vi "4461.Trigger.vi"(8 "error in (no error)":errorcluster, 11 "Instrument.Lockin in":refnum<class "Instrument.Lockin.lvclass">) -> (0 "error out":errorcluster, 3 "Instrument.Lockin out":refnum<class "Instrument.Lockin.lvclass">)   [LabVIEW 2016, in "LockinDAQ.lvclass"]
uses:
  LockinDAQ.lvclass
  <resource>/objmgr/daqmx.rc
  Typedefs/DAQType-enum.ctl
  <vilib>/DAQmx/configure/trigger.llb/DAQmx Start Trigger (Digital Edge).vi
  Instrument.Lockin/Instrument.Lockin.lvclass
  C:/Program Files (x86)/National Instruments/LabVIEW 2016/user.lib/LevyLab/Levylab Instruments/SMOs/Instrument/Instrument.lvclass
  C:/Program Files (x86)/National Instruments/LabVIEW 2016/user.lib/LevyLab/Levylab Instruments/SMOs/LevyLab/LevyLab.lvclass
  C:/Program Files (x86)/National Instruments/LabVIEW 2016/vi.lib/JKI/JKI SMO/SMO/SMO.lvclass
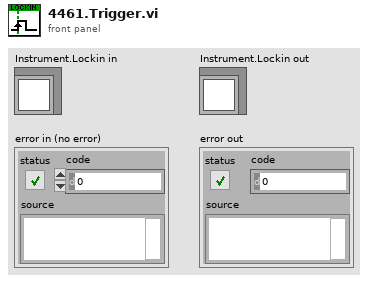
[diagram p1: front panel]
types:
  T1 = typedef "LockinDAQ.lvclass/DAQType-enum.ctl" = enum16{"None", "USB 4431", "PXI 446x"}
  T2 = cluster{"DAQ Type":T1, "master task":refnum<k21>, "RefClk.Src":tag, "SyncPulse.Src":tag, "Trigger.Src":tag, "SyncPulse.SyncTime":dbl}
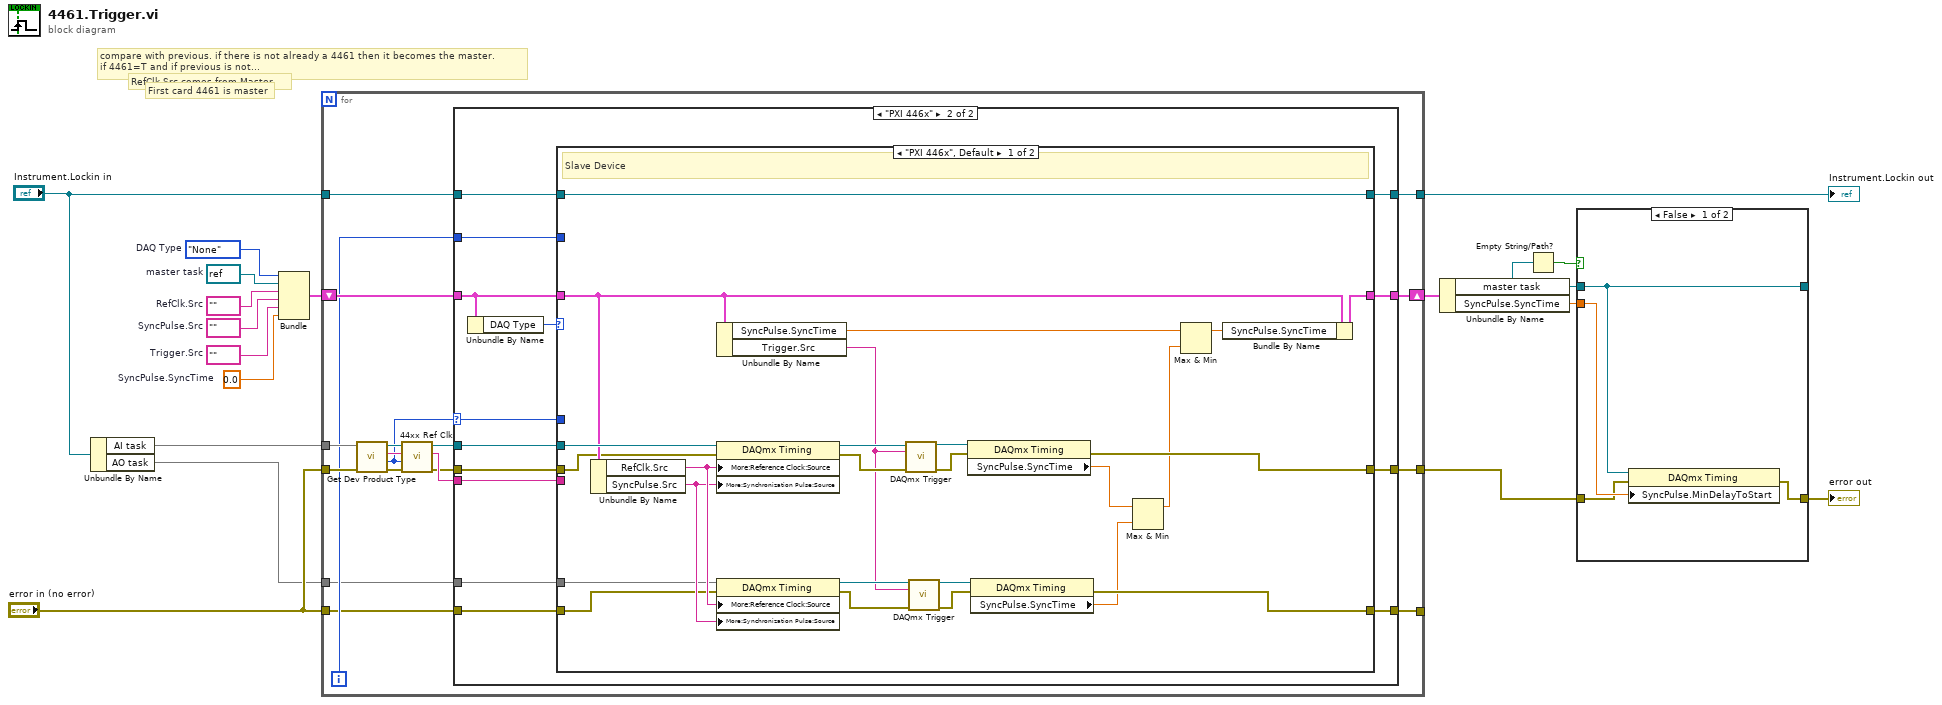
[diagram p0: block diagram]
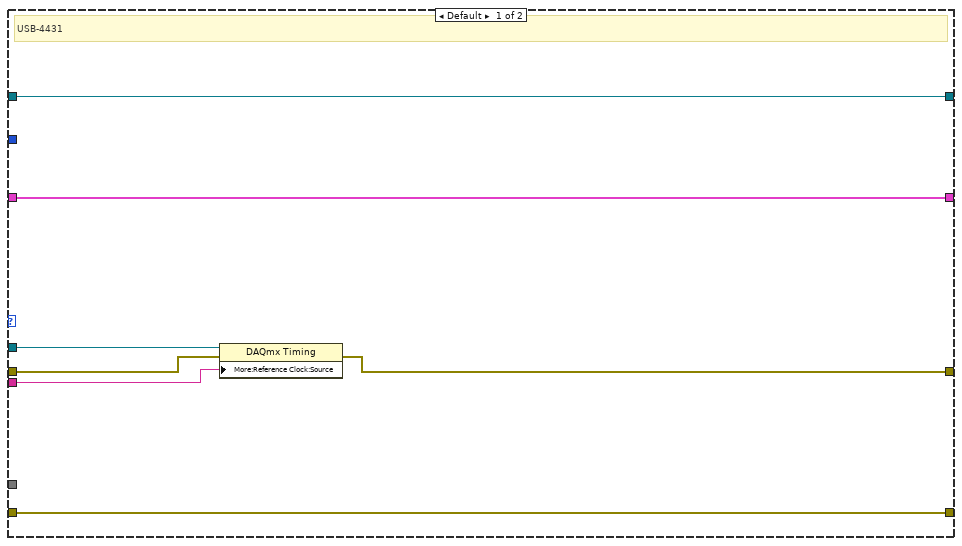
[diagram p2: hidden frame]
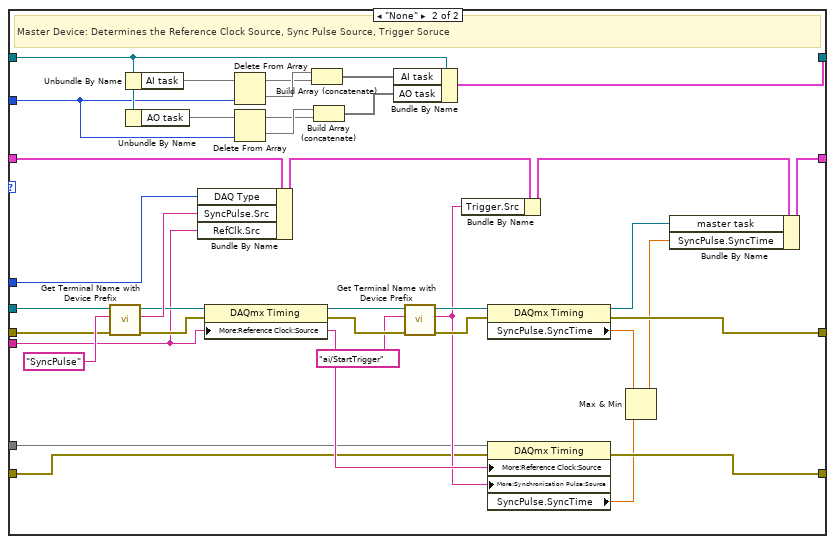
[diagram p3: hidden frame]
diagram:
  w2 = refnum<k21> refnum  # master task
  w12 = 0.0  # SyncPulse.SyncTime
  w11 = tag ""  # Trigger.Src
  w10 = tag ""  # SyncPulse.Src
  w3 = tag ""  # RefClk.Src
  w1 = DAQType-enum."None"  # DAQ Type
  # "RefClk.Src comes from Master"
  # "compare with previous. if there is not already a 4461 then it becomes the master. \nif 4461=T and if previous is not..."
  # "First card 4461 is master"
  n1 = Unbundle By Name("Instrument.Lockin in") -> ("AI task"=w6, "AO task"=w4)
  n2 = Bundle("DAQ Type"=w1, "master task"=w2, "RefClk.Src"=w3, "SyncPulse.Src"=w10, "Trigger.Src"=w11, "SyncPulse.SyncTime"=w12) -> (w9:T2)  [unwired: 1 in]
  n3 = for {
    tunnel: w6 -> [w36]
    tunnel: "error in (no error)" -> [w32]
    shift-right: [w27] -> w13
    shift-left: w9 -> [w30]
    tunnel: [w25] -> w17
    tunnel: "Instrument.Lockin in" -> [w24]
    tunnel: [w22] -> w7
    tunnel: [w21] -> _
    tunnel: "error in (no error)" -> [w20]
    tunnel: w4 -> [w19]
    i -> [w23]
    n4 = call "Get Dev Product Type.vi"("error in (no error)"=w32, "Refnum in"=w36) -> ("error out"=w35:errorcluster, "DAQ Type"=w31:T1, "ActiveDev"=w34:tag, "Refnum out"=w33:refnum<k21>)  [unwired: 6 in]
    n5 = call "44xx Ref Clk.vi"("error in (no error)"=w35, "DAQ Type"=w31, "ActiveDev"=w34, "Refnum in"=w33) -> ("error out"=w26:errorcluster, "RefClk.Src"=w28:tag, "Refnum out"=w29:refnum<k21>)  [unwired: 5 in]
    n6 = case shown="\"PXI 446x\"" w31 {
      selector: w31 -> [_ w54]
      tunnel: w30 -> [w43 w55]
      tunnel: w29 -> [w42 w57]
      tunnel: w28 -> [w41 w56]
      tunnel: [w43 w53] -> w27
      tunnel: w26 -> [w40 w52]
      tunnel: [w39 w51] -> w25
      tunnel: w24 -> [w38 w49]
      tunnel: w23 -> [_ w48]
      tunnel: [w38 w47] -> w22
      tunnel: [w37 w44] -> w21
      tunnel: w20 -> [w37 w46]
      tunnel: w19 -> [_ w45]
      frame Default {
        # "USB-4431"
        n7 = property class="DAQmx Timing"(reference=w42, error in=w40, "More:Reference Clock:Source"=w41) -> (error out=w39:errorcluster)  [unwired: 1 out]
      }
      frame "PXI 446x" {
        n8 = Unbundle By Name(w55) -> ("DAQ Type"=w50:T1)
        n9 = case shown="\"PXI 446x\", Default" w50 {
          tunnel: w57 -> [w82 w119]
          tunnel: w56 -> [_ w96]
          tunnel: w55 -> [w79 w118]
          tunnel: w54 -> [_ w117]
          tunnel: [w78 w106] -> w53
          tunnel: w52 -> [w65 w114]
          tunnel: [w76 w105] -> w51
          tunnel: w49 -> [w75 w91]
          tunnel: w48 -> [_ w90]
          tunnel: [w75 w97] -> w47
          tunnel: w46 -> [w64 w93]
          tunnel: w45 -> [w72 w94]
          tunnel: [w63 w92] -> w44
          frame "PXI 446x", Default {
            # "Slave Device"
            n10 = Unbundle By Name(w79) -> ("RefClk.Src"=w74:tag, "SyncPulse.Src"=w73:tag)
            n11 = Unbundle By Name(w79) -> ("SyncPulse.SyncTime"=w60:dbl, "Trigger.Src"=w68:tag)
            n12 = property class="DAQmx Timing"(reference=w82, error in=w65, "More:Reference Clock:Source"=w74, "More:Synchronization Pulse:Source"=w73) -> (reference out=w81:refnum<k21>, error out=w69:errorcluster)
            n13 = property class="DAQmx Timing"(reference=w72, error in=w64, "More:Reference Clock:Source"=w74, "More:Synchronization Pulse:Source"=w73) -> (reference out=w70:refnum<k21>, error out=w67:errorcluster)
            n14 = call-poly <vilib>:"DAQmx Trigger.vi"("task/channels in"=w81, "source"=w68, "error in"=w69) -> ("task out"=w80:refnum<k21>, "error out"=w77:errorcluster)  [unwired: 11 in]
            n15 = call-poly <vilib>:"DAQmx Trigger.vi"("task/channels in"=w70, "source"=w68, "error in"=w67) -> ("task out"=w71:refnum<k21>, "error out"=w66:errorcluster)  [unwired: 11 in]
            n16 = property class="DAQmx Timing"(reference=w80, error in=w77) -> (error out=w76:errorcluster, "SyncPulse.SyncTime"=w58:dbl)  [unwired: 1 out]
            n17 = property class="DAQmx Timing"(reference=w71, error in=w66) -> (error out=w63:errorcluster, "SyncPulse.SyncTime"=w62:dbl)  [unwired: 1 out]
            n18 = Max & Min(x=w58, y=w62) -> (max(x,y)=w61:dbl)  [unwired: 1 out]
            n19 = Max & Min(x=w60, y=w61) -> (max(x,y)=w59:dbl)  [unwired: 1 out]
            n20 = Bundle By Name(cluster=w79, "SyncPulse.SyncTime"=w59) -> (w78:T2)
          }
          frame "None" {
            # "Master Device: Determines the Reference Clock Source, Sync Pulse Source, Trigger Soruce"
            n21 = call "Get Terminal Name with Device Prefix.vi"("error in (no error)"=w114, "Local Terminal Name"="SyncPulse", "task/channels in"=w119) -> ("error out"=w113:errorcluster, "Terminal Name with Device Prefix"=w115:tag, "task out"=w103:refnum<k21>)  [unwired: 6 in]
            n22 = Unbundle By Name(w91) -> ("AI task"=w101)
            n23 = Unbundle By Name(w91) -> ("AO task"=w89)
            n24 = Bundle By Name(cluster=w118, "DAQ Type"=w117, "SyncPulse.Src"=w115, "RefClk.Src"=w96) -> (w109:T2)
            n25 = property class="DAQmx Timing"(reference=w103, error in=w113, "More:Reference Clock:Source"=w96) -> (reference out=w110:refnum<k21>, error out=w112:errorcluster)
            n26 = Delete From Array(array=w101, index=w90) -> (deleted portion=w100, array with subset deleted=w99)  [unwired: 1 in]
            n27 = Delete From Array(array=w89, index=w90) -> (deleted portion=w88, array with subset deleted=w87)  [unwired: 1 in]
            n28 = Build Array (concatenate)(w100, w99) -> (w98:void[])
            n29 = Build Array (concatenate)(w88, w87) -> (w86:void[])
            n30 = Bundle By Name(cluster=w91, "AI task"=w98, "AO task"=w86) -> (w97:cluster{})
            n31 = call "Get Terminal Name with Device Prefix.vi"("error in (no error)"=w112, "Local Terminal Name"="ai/StartTrigger", "task/channels in"=w110) -> ("error out"=w107:errorcluster, "Terminal Name with Device Prefix"=w95:tag, "task out"=w108:refnum<k21>)  [unwired: 6 in]
            n32 = Bundle By Name(cluster=w109, "Trigger.Src"=w95) -> (w104:T2)
            n33 = property class="DAQmx Timing"(reference=w108, error in=w107) -> (reference out=w102:refnum<k21>, error out=w105:errorcluster, "SyncPulse.SyncTime"=w85:dbl)
            n34 = property class="DAQmx Timing"(reference=w94, error in=w93, "More:Reference Clock:Source"=w96, "More:Synchronization Pulse:Source"=w95) -> (error out=w92:errorcluster, "SyncPulse.SyncTime"=w84:dbl)  [unwired: 1 out]
            n35 = Max & Min(x=w85, y=w84) -> (max(x,y)=w83:dbl)  [unwired: 1 out]
            n36 = Bundle By Name(cluster=w104, "master task"=w102, "SyncPulse.SyncTime"=w83) -> (w106:T2)
          }
        }
      }
    }
  }
  "Instrument.Lockin out" <- w7
  n37 = Unbundle By Name(w13) -> ("master task"=w15:refnum<k21>, "SyncPulse.SyncTime"=w16:dbl)
  n38 = Empty String/Path?(string/path=w15) -> (empty?=w14:bool)
  n39 = case shown="False" w14 {
    tunnel: w15 -> [w120 w124]
    tunnel: w16 -> [w123 _]
    tunnel: w17 -> [w122 w125]
    tunnel: [w121 w125] -> w18
    tunnel: [w120 w124] -> _
    frame False {
      n40 = property class="DAQmx Timing"(reference=w120, error in=w122, "SyncPulse.MinDelayToStart"=w123) -> (error out=w121:errorcluster)  [unwired: 1 out]
    }
    frame True {
      # "If master task=empty, then no master devices were ever found (ie, all 4431s)"
    }
  }
  "error out" <- w18
